vi "Main.vi"() -> ()   [LabVIEW 2010]
uses:
  Ctrls/Main_states.ctl
  Ctrls/Main_Msg_type.ctl
  Ctrls/NS3_commands.ctl
  Ctrls/ODSS_Msgs.ctl
  Vars/Comm_Vars.vi
panel:
  out "Time":timestamp caption="Simulation Time" format="%<%H:%M>T"
  out "V2":T1(graph) caption="Meter M2"
  out "Data":bool
  out "M2":string[][](table) caption="Monitor M2"
  out "M1":string[][](table) caption="Monitor M1"
  out "V1":T1(graph) caption="Meter M1"
  in  "ODSS Step":dbl[][](array[numeric])
  in  "NS3 Step":dbl[](array[numeric])
  out "Status":string
  in  "Stop":bool
  in  "Tasks":bool[](array[boolean])
  out "error out":errorcluster
  out "GB":picture
  in  "Quit":bool
  in  "start":bool
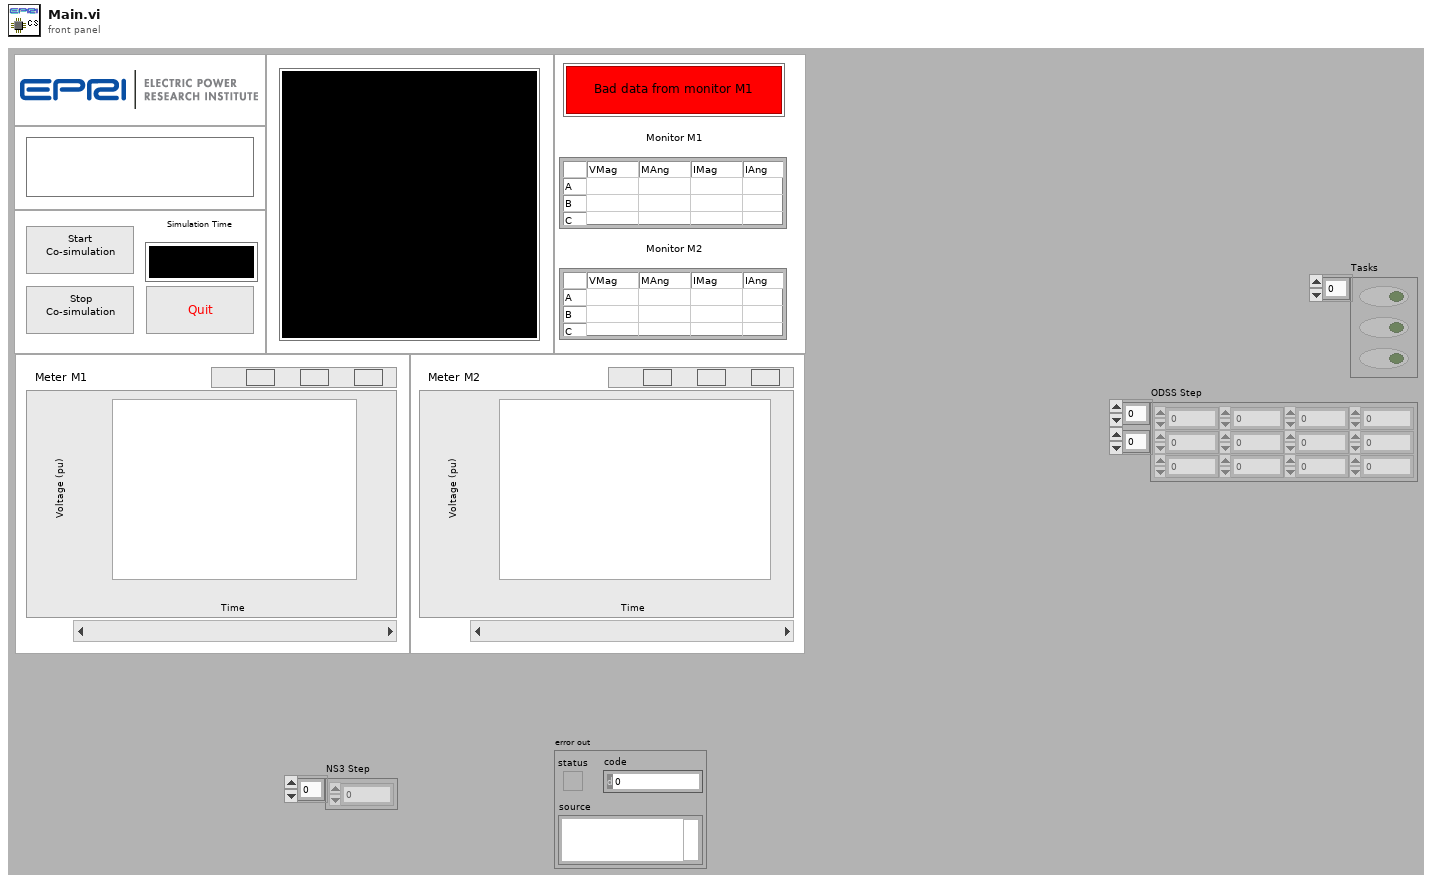
[diagram p1: front panel]
types:
  T1 = cluster{"Numeric":dbl, "Numeric":dbl, "Numeric":dbl}
  T2 = typedef "Main_Msg_type.ctl" = enum16{"Task end", "NS3 ready", "NS3 data", "Meter data", "exit"}
  T3 = typedef "Main_states.ctl" = enum16{"Init", "Launch NS3", "Launch OpenDSS", "Launch Meters", "Wait 4 user input", "Simulate", "Step in NS3", "Step in OpenDSS", "Publish Data", "Wait 4 Actors", "Kill actors", "Start exit routine", "Paint Meters", "End"}
  T4 = cluster{"Main_States":T3, "queue":refnum<queue>, "exit":bool, "Sim Started":bool, "Status":string, "next state":T3, "Bus info":cluster{"Bus Names":string[], "Bus Coords":cluster{i32, i32}[]}, "Circuit":picture, "Sim time":i32, "Paint":bool}
  T5 = cluster{"Rotate 90 deg":bool, "Flip Horizontally":bool, "Flip vertically":bool}
  T6 = cluster{"actor_name":string, "actor_type":string, "queue":refnum<queue>}[]
  T7 = typedef "NS3_commands.ctl" = enum16{"Init NS3 Sim", "Step in", "Exit"}
  T8 = typedef "ODSS_Msgs.ctl" = enum16{"Step in", "Exit", "Sim Time", "Set Working Dir"}
  T9 = cluster{"Numeric":dbl, "Numeric":dbl, "Numeric":dbl}[]
  T10 = cluster{"Bus Names":string[], "Bus Coords":cluster{i32, i32}[]}
  T11 = typedef "LVDateTimeRec.ctl" = cluster{"fractional second":dbl, "second":i32, "minute":i32, "hour":i32, "day of month":i32, "month":i32, "year":i32, "day of week":i32, "day of year":i32, "DST":i32}
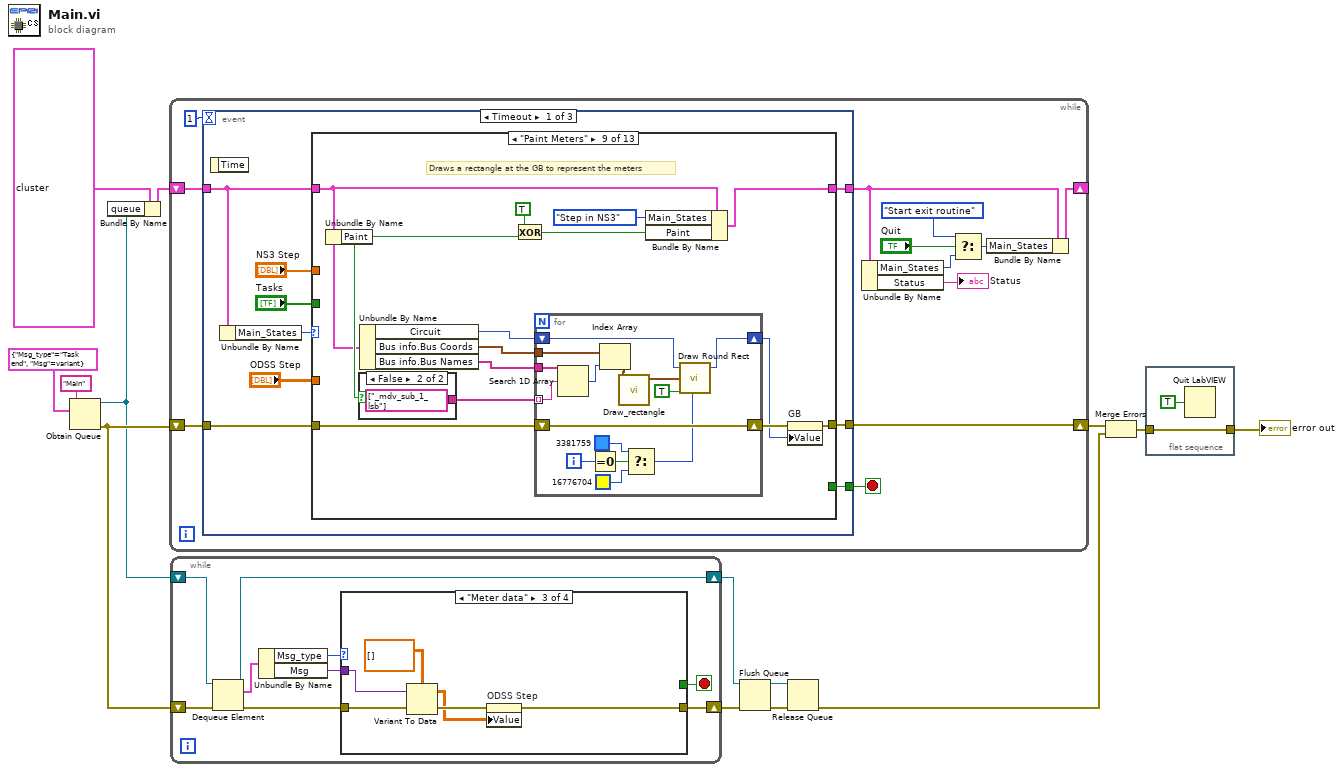
[diagram p0: block diagram]
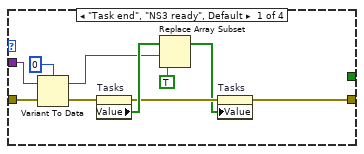
[diagram p2: hidden frame]
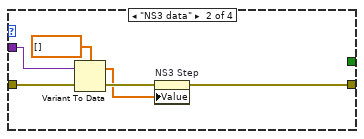
[diagram p3: hidden frame]
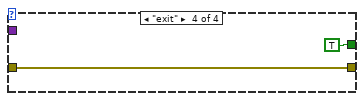
[diagram p4: hidden frame]
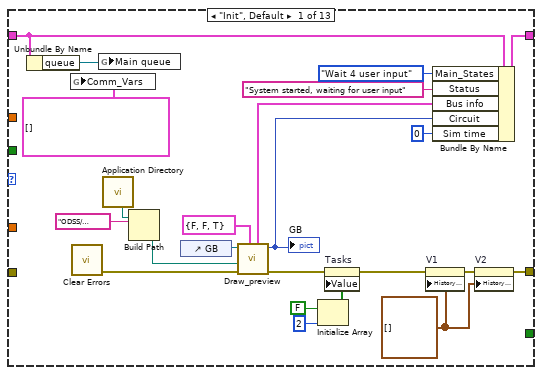
[diagram p5: hidden frame]
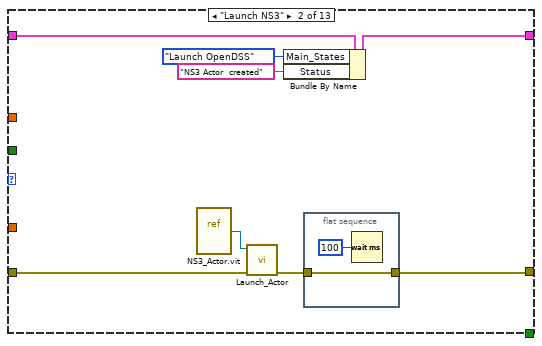
[diagram p6: hidden frame]
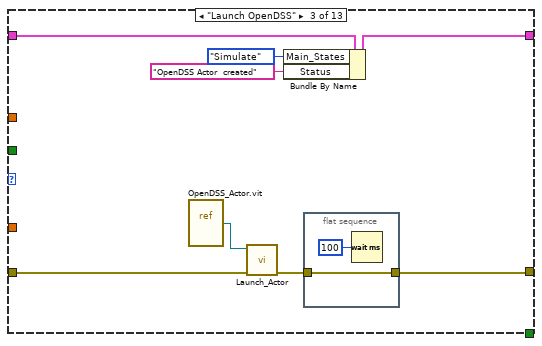
[diagram p7: hidden frame]
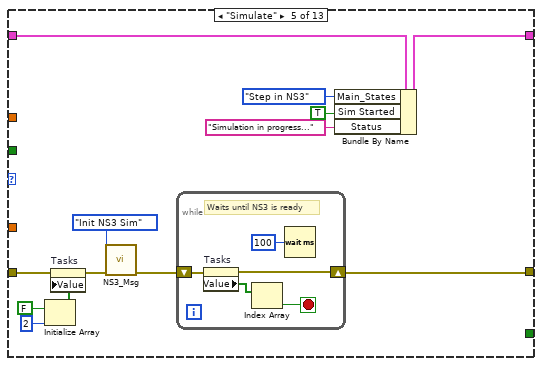
[diagram p9: hidden frame]
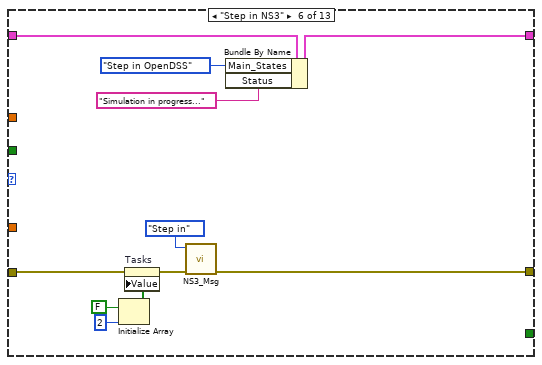
[diagram p10: hidden frame]
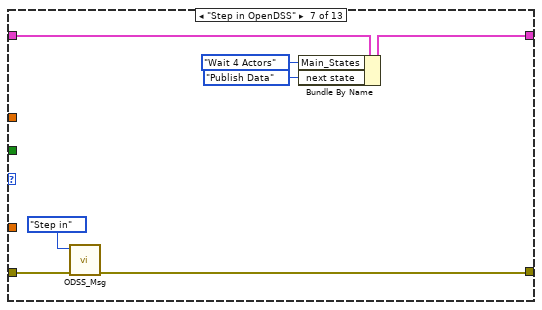
[diagram p11: hidden frame]
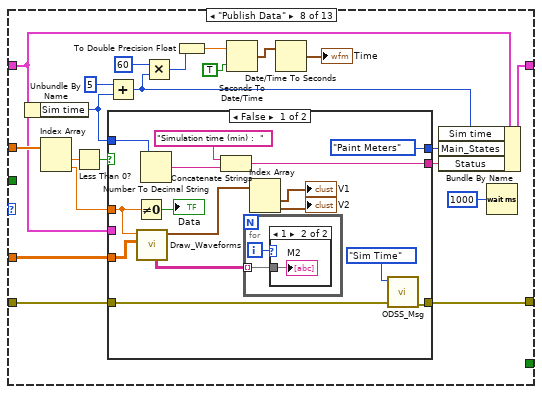
[diagram p12: hidden frame]
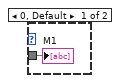
[diagram p13: hidden frame]
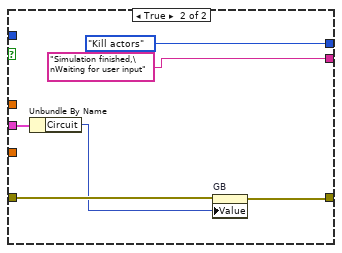
[diagram p14: hidden frame]
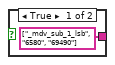
[diagram p15: hidden frame]
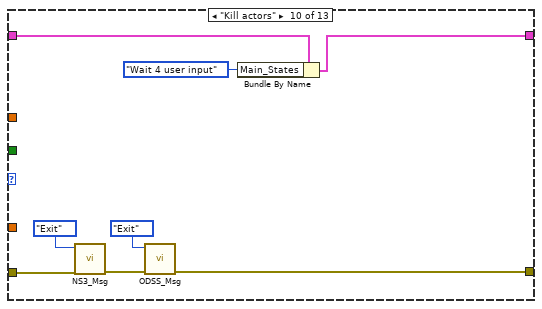
[diagram p16: hidden frame]
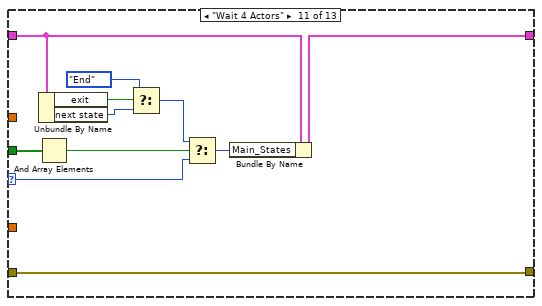
[diagram p17: hidden frame]
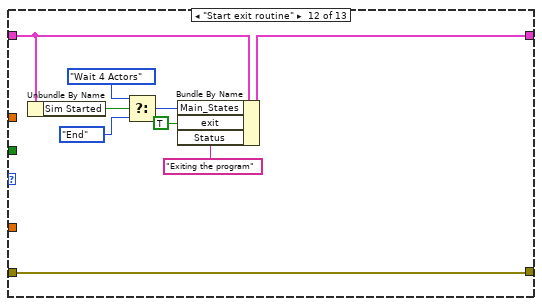
[diagram p18: hidden frame]
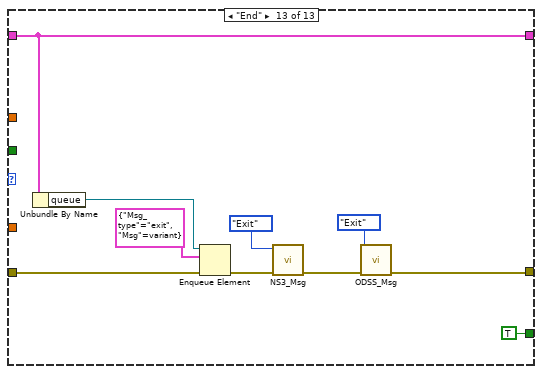
[diagram p19: hidden frame]
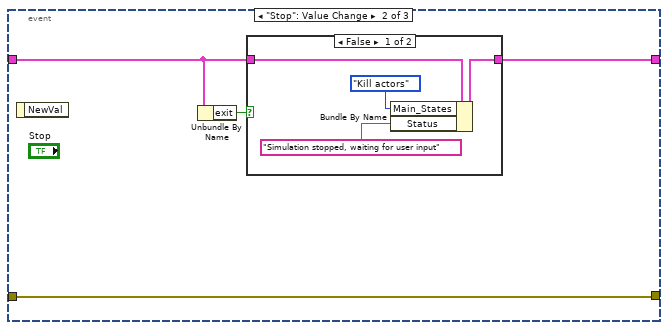
[diagram p20: hidden frame]
diagram:
  n1 = Obtain Queue(name (unnamed)="Main", element data type=cluster{"Msg_type":T2, "Msg":variant} {"Msg_type"=enum."Task end", "Msg"=variant}) -> (queue out=w10:refnum<queue>, error out=w12:errorcluster)  [unwired: 3 in, 1 out]
  n2 = Bundle By Name(cluster=T4 {"Main_States"=enum."Init", "queue"=refnum, "exit"=FALSE, "Sim Started"=FALSE, "Status"="", "next state"=enum."Init", "Bus info"={"Bus Names"=[], "Bus Coords"=[]}, "Circuit"=bytes[32946], "Sim time"=0, "Paint"=FALSE} ("variables"), "queue"=w10) -> (w3:T4)
  n3 = while {
    shift-right: [w16] -> _
    shift-left: w3 -> [w25]
    shift-right: [w23] -> w5
    shift-left: w12 -> [w22]
    stop <- w24 stop-if-true
    n4 = event shown="[0] Timeout" {
      selector: _ -> [_ _ _]
      dyn-events: _ -> [_ _ _]
      timeout: 1 -> [_ _ _]
      tunnel: w25 -> [w34 w234 w244]
      tunnel: [w33 w233 w242] -> w18
      tunnel: [w32 _ _] -> w24
      tunnel: [w27 w235 w245] -> w23
      tunnel: w22 -> [w31 w235 w245]
      event Timeout {
        n5 = event-data() -> ()  [unwired: 1 in, 1 out]
        n6 = Unbundle By Name(w34) -> ("Main_States"=w35:T3)
        n7 = case shown="\"Paint Meters\"" w35 {
          selector: w35 -> [_ _ _ _ _ _ _ _ _ _ w210 _ _]
          tunnel: w34 -> [w47 w65 w75 w80 w93 w105 w114 w117 w166 w201 w207 w219 w230]
          tunnel: [w56 w63 w73 w80 w92 w103 w113 w129 w175 w200 w208 w220 w230] -> w33
          tunnel: [_ _ _ _ _ _ _ _ _ _ _ _ TRUE] -> w32
          tunnel: w31 -> [_ w66 w76 w79 w86 w102 w116 w126 w169 w197 w202 w213 w227]
          tunnel: "Tasks" -> [_ _ _ _ _ _ _ _ _ _ w212 _ _]
          tunnel: "NS3 Step" -> [_ _ _ _ _ _ _ w128 _ _ _ _ _]
          tunnel: "ODSS Step" -> [_ _ _ _ _ _ _ w127 _ _ _ _ _]
          tunnel: [w38 w60 w70 w79 w81 w99 w110 w125 w171 w194 w202 w213 w223] -> w27
          frame "Init", Default {
            w37 = T9 [] ("History Data")
            n8 = Unbundle By Name(w47) -> ("queue"=w46:refnum<queue>)
            n9 = global write "Comm_Vars.vi" "Comm_Vars"(T6 [] ("Comm_Vars")) -> ()
            n10 = call <vilib>:"Clear Errors.vi"() -> ("error out"=w54:errorcluster)  [unwired: 7 in]
            n11 = global write "Comm_Vars.vi" "Main queue"(w46) -> ()
            n12 = call <vilib>:"Application Directory.vi"() -> ("Application Directory"=w52:path)
            n13 = Build Path(base path=w52, name or relative path="ODSS/BusCoords.dss") -> (appended path=w50:path)
            n14 = control-ref of="GB"() -> (w55:refnum<vi>)
            n15 = call "Draw_preview.vi"("Draw_ops"=T5 {"Rotate 90 deg"=FALSE, "Flip Horizontally"=FALSE, "Flip vertically"=TRUE}, "error in (no error)"=w54, "Path"=w50, "Picture ref"=w55) -> ("error out"=w45:errorcluster, "Picture out"=w41:picture, "Bus info"=w42:T10)  [unwired: 5 in]
            "GB" <- w41
            n16 = Initialize Array(FALSE, 2 ("dimension size")) -> (w44:bool[])
            n17 = property on="Tasks" class="Arr (strict)"(error in=w45, "Value"=w44) -> (error out=w36:errorcluster)  [unwired: 1 in, 1 out]
            n18 = property on="V1" class="WFChart (strict)"(error in=w36, "History Data"=w37) -> (error out=w39:errorcluster)  [unwired: 1 in, 1 out]
            n19 = Bundle By Name(cluster=w47, "Main_States"=Main_states."Wait 4 user input", "Status"="System started, waiting for user input", "Bus info"=w42, "Circuit"=w41, "Sim time"=0) -> (w56:T4)
            n20 = property on="V2" class="WFChart (strict)"(error in=w39, "History Data"=w37) -> (error out=w38:errorcluster)  [unwired: 1 in, 1 out]
          }
          frame "Launch NS3" {
            n21 = vi-ref "NS3_Actor.vit"() -> (w59:refnum<vi>)
            n22 = call "Launch_Actor.vi"("error in"=w66, "vi reference"=w59) -> ("error out"=w61:errorcluster)  [unwired: 9 in]
            n23 = Bundle By Name(cluster=w65, "Main_States"=Main_states."Launch OpenDSS", "Status"="NS3 Actor  created") -> (w63:T4)
            n24 = flat-sequence {
              tunnel: w61 -> [w68]
              tunnel: [w68] -> w60
              frame #0 {
                n25 = Wait (ms)(milliseconds to wait=u32 100) -> ()  [unwired: 1 out]
              }
            }
          }
          frame "Launch OpenDSS" {
            n26 = vi-ref "OpenDSS_Actor.vit"() -> (w69:refnum<vi>)
            n27 = call "Launch_Actor.vi"("error in"=w76, "vi reference"=w69) -> ("error out"=w71:errorcluster)  [unwired: 9 in]
            n28 = Bundle By Name(cluster=w75, "Main_States"=Main_states."Simulate", "Status"="OpenDSS Actor  created") -> (w73:T4)
            n29 = flat-sequence {
              tunnel: w71 -> [w78]
              tunnel: [w78] -> w70
              frame #0 {
                n30 = Wait (ms)(milliseconds to wait=u32 100) -> ()  [unwired: 1 out]
              }
            }
          }
          frame "Wait 4 user input" {
          }
          frame "Simulate" {
            n31 = Initialize Array(FALSE, 2 ("dimension size")) -> (w87:bool[])
            n32 = property on="Tasks" class="Arr (strict)"(error in=w86, "Value"=w87) -> (error out=w85:errorcluster)  [unwired: 1 in, 1 out]
            n33 = call "NS3_Msg.vi"("error in"=w85, "Msg"=NS3_commands."Init NS3 Sim") -> ("error out"=w82:errorcluster)  [unwired: 9 in]
            n34 = while {
              shift-right: [w97] -> w81
              shift-left: w82 -> [w98]
              stop <- w95 stop-if-true
              # "Waits until NS3 is ready"
              n35 = property on="Tasks" class="Arr (strict)"(error in=w98) -> (error out=w97:errorcluster, "Value"=w96:bool[])  [unwired: 1 in, 1 out]
              n36 = Index Array(array=w96) -> (element=w95:bool)  [unwired: 1 in]
              n37 = Wait (ms)(milliseconds to wait=u32 100) -> ()  [unwired: 1 out]
            }
            n38 = Bundle By Name(cluster=w93, "Main_States"=Main_states."Step in NS3", "Sim Started"=TRUE, "Status"="Simulation in progress...") -> (w92:T4)
          }
          frame "Step in NS3" {
            n39 = Initialize Array(FALSE, 2 ("dimension size")) -> (w106:bool[])
            n40 = property on="Tasks" class="Arr (strict)"(error in=w102, "Value"=w106) -> (error out=w101:errorcluster)  [unwired: 1 in, 1 out]
            n41 = call "NS3_Msg.vi"("error in"=w101, "Msg"=NS3_commands."Step in") -> ("error out"=w99:errorcluster)  [unwired: 9 in]
            n42 = Bundle By Name(cluster=w105, "Main_States"=Main_states."Step in OpenDSS", "Status"="Simulation in progress...") -> (w103:T4)
          }
          frame "Step in OpenDSS" {
            n43 = call "ODSS_Msg.vi"("error in"=w116, "Msg"=ODSS_Msgs."Step in") -> ("error out"=w110:errorcluster)  [unwired: 9 in]
            n44 = Bundle By Name(cluster=w114, "Main_States"=Main_states."Wait 4 Actors", "next state"=Main_states."Publish Data") -> (w113:T4)
          }
          frame "Publish Data" {
            n45 = Unbundle By Name(w117) -> ("Sim time"=w131:i32)
            n46 = Index Array(array=w128) -> (element #1=w135:dbl, element #2=w132:dbl)  [unwired: 2 in]
            n47 = Less Than 0?(x=w135) -> (x < 0?=w136:bool)
            n48 = Add(x=5, y=w131) -> (x+y=w124:i32)
            n49 = case shown="False" w136 {
              tunnel: w131 -> [w151 _]
              tunnel: [Main_states."Paint Meters" ("Main_States") Main_states."Kill actors" ("t")] -> w134
              tunnel: [w148 "Simulation finished,\nWaiting for user input" ("Status")] -> w133
              tunnel: w132 -> [w141 _]
              tunnel: w127 -> [w147 _]
              tunnel: w126 -> [w139 w160]
              tunnel: [w143 w159] -> w125
              tunnel: w117 -> [_ w158]
              frame False {
                n50 = Not Equal To 0?(x=w141) -> (x != 0?=→"Data":bool)
                n51 = call "Draw_Waveforms.vi"("ODSS Step"=w147, "Comm"=w141) -> ("Time M"=w146:T9, "Meter"=w140:string[][][])  [unwired: 8 in]
                n52 = Number To Decimal String(number=w151) -> (decimal integer string=w149:string)  [unwired: 1 in]
                n53 = Concatenate Strings("Simulation time (min) :  ", w149) -> (w148:string)
                n54 = for {
                  tunnel: w140 -> [w153] mode=indexing
                  i -> [w154]
                  n55 = case shown="1" w154 {
                    tunnel: w153 -> [w155 w156]
                    frame 0, Default {
                      "M1" <- w155
                    }
                    frame 1 {
                      "M2" <- w156
                    }
                  }
                }
                n56 = Index Array(array=w146) -> (element #1=→"V1":T1, element #2=→"V2":T1)  [unwired: 2 in]
                n57 = call "ODSS_Msg.vi"("error in"=w139, "Msg"=ODSS_Msgs."Sim Time") -> ("error out"=w143:errorcluster)  [unwired: 9 in]
              }
              frame True {
                n58 = Unbundle By Name(w158) -> ("Circuit"=w157:picture)
                n59 = property on="GB" class="Pict"(error in=w160, "Value"=w157) -> (error out=w159:errorcluster)  [unwired: 1 in, 1 out]
              }
            }
            n60 = Multiply(x=60, y=w124) -> (x*y=w122:i32)
            n61 = To Double Precision Float(number=w122) -> (double precision float=w121:dbl)
            n62 = Seconds To Date/Time(time stamp (now)=w121, to UTC (F)=TRUE) -> (date time rec=w120:T11)
            n63 = Date/Time To Seconds(2:w120) -> (0:→"Time":timestamp)  [unwired: 1 in]
            n64 = Bundle By Name(cluster=w117, "Sim time"=w124, "Main_States"=w134, "Status"=w133) -> (w129:T4)
            n65 = Wait (ms)(milliseconds to wait=u32 1000) -> ()  [unwired: 1 out]
          }
          frame "Paint Meters" {
            # "Draws a rectangle at the GB to represent the meters"
            n66 = Unbundle By Name(w166) -> ("Paint"=w172:bool)
            n67 = case shown="False" w172 {
              tunnel: [string[] ["_mdv_sub_1_lsb", "6580", "69490"] string[] ["_mdv_sub_1_lsb"]] -> w167
              frame True {
              }
              frame False {
              }
            }
            n68 = Unbundle By Name(w166) -> ("Circuit"=w163:picture, "Bus info.Bus Coords"=w164:cluster{i32, i32}[], "Bus info.Bus Names"=w165:string[])
            n69 = Exclusive Or(1:w172, 2:TRUE ("x")) -> (0:w173:bool)
            n70 = for {
              shift-right: [w188] -> w170
              shift-left: w169 -> [w188]
              tunnel: w165 -> [w191]
              tunnel: w164 -> [w190]
              shift-right: [w186] -> w168
              shift-left: w163 -> [w187]
              tunnel: w167 -> [w177] mode=indexing
              i -> [w182]
              n71 = Search 1D Array(1D array=w191, element=w177) -> (index of element=w189:i32)  [unwired: 1 in]
              n72 = Equal To 0?(x=w182) -> (x = 0?=w181:bool)
              n73 = Index Array(array=w190, index=w189) -> (element=w185:cluster{i32, i32})
              n74 = call "Draw_rectangle.vi"("Coords"=w185) -> ("rect"=w184:cluster{i32, i32, i32, i32})  [unwired: 10 in]
              n75 = Select(t=u32 3381759 ("color(black)"), s=w181, f=u32 16776704 ("color(black)")) -> (s? t:f=w178:u32)
              n76 = call <vilib>:"Draw Round Rect.vi"("picture"=w187, "rect"=w184, "fill?(F)"=TRUE, "color(black)"=w178) -> ("new picture"=w186:picture)  [unwired: 5 in]
            }
            n77 = Bundle By Name(cluster=w166, "Main_States"=Main_states."Step in NS3", "Paint"=w173) -> (w175:T4)
            n78 = property on="GB" class="Pict"(error in=w170, "Value"=w168) -> (error out=w171:errorcluster)  [unwired: 1 in, 1 out]
          }
          frame "Kill actors" {
            n79 = call "NS3_Msg.vi"("error in"=w197, "Msg"=NS3_commands."Exit") -> ("error out"=w195:errorcluster)  [unwired: 9 in]
            n80 = call "ODSS_Msg.vi"("error in"=w195, "Msg"=ODSS_Msgs."Exit") -> ("error out"=w194:errorcluster)  [unwired: 9 in]
            n81 = Bundle By Name(cluster=w201, "Main_States"=Main_states."Wait 4 user input") -> (w200:T4)
          }
          frame "Wait 4 Actors" {
            n82 = Unbundle By Name(w207) -> ("exit"=w206:bool, "next state"=w203:T3)
            n83 = And Array Elements(Boolean array=w212) -> (logical AND=w211:bool)
            n84 = Select(t=Main_states."End", s=w206, f=w203) -> (s? t:f=w204:T3)
            n85 = Select(t=w204, s=w211, f=w210) -> (s? t:f=w209:T3)
            n86 = Bundle By Name(cluster=w207, "Main_States"=w209) -> (w208:T4)
          }
          frame "Start exit routine" {
            n87 = Unbundle By Name(w219) -> ("Sim Started"=w218:bool)
            n88 = Select(t=Main_states."Wait 4 Actors" ("Main_States"), s=w218, f=Main_states."End" ("Main_States")) -> (s? t:f=w215:T3)
            n89 = Bundle By Name(cluster=w219, "Main_States"=w215, "exit"=TRUE, "Status"="Exiting the program") -> (w220:T4)
          }
          frame "End" {
            n90 = Unbundle By Name(w230) -> ("queue"=w229:refnum<queue>)
            n91 = Enqueue Element(queue=w229, element=cluster{"Msg_type":T2, "Msg":variant} {"Msg_type"=enum."exit", "Msg"=variant}, error in (no error)=w227) -> (error out=w225:errorcluster)  [unwired: 1 in, 2 out]
            n92 = call "NS3_Msg.vi"("error in"=w225, "Msg"=NS3_commands."Exit") -> ("error out"=w224:errorcluster)  [unwired: 9 in]
            n93 = call "ODSS_Msg.vi"("error in"=w224, "Msg"=ODSS_Msgs."Exit") -> ("error out"=w223:errorcluster)  [unwired: 9 in]
          }
        }
      }
      event "Stop": Value Change {
        n94 = event-data() -> ()  [unwired: 1 in, 1 out]
        n95 = Unbundle By Name(w234) -> ("exit"=w232:bool)
        n96 = case shown="False" w232 {
          tunnel: w234 -> [w239 w240]
          tunnel: [w238 w240] -> w233
          frame False {
            n97 = Bundle By Name(cluster=w239, "Main_States"=Main_states."Kill actors" ("f"), "Status"="Simulation stopped, waiting for user input") -> (w238:T4)
          }
          frame True {
          }
        }
      }
      event "start": Value Change {
        n98 = event-data() -> ()  [unwired: 1 in, 1 out]
        n99 = Bundle By Name(cluster=w244, "Main_States"=Main_states."Launch NS3", "Status"="Initializing simulation") -> (w242:T4)
      }
    }
    n100 = Unbundle By Name(w18) -> ("Main_States"=w20:T3, "Status"=→"Status":string)
    n101 = Select(t=Main_states."Start exit routine" ("Main_States"), s="Quit", f=w20) -> (s? t:f=w17:T3)
    n102 = Bundle By Name(cluster=w18, "Main_States"=w17) -> (w16:T4)
  }
  n103 = while {
    shift-right: [w249] -> w9
    shift-left: w12 -> [w254]
    shift-right: [w246] -> w8
    shift-left: w10 -> [w247]
    stop <- w248 stop-if-true
    n104 = Dequeue Element(queue=w247, error in (no error)=w254) -> (queue out=w246:refnum<queue>, element=w253:cluster{"Msg_type":T2, "Msg":variant}, error out=w250:errorcluster)  [unwired: 1 in, 1 out]
    n105 = Unbundle By Name(w253) -> ("Msg_type"=w252:T2, "Msg"=w251:variant)
    n106 = case shown="\"Meter data\"" w252 {
      tunnel: w251 -> [w263 w269 w275 _]
      tunnel: w250 -> [w264 w270 w276 w278]
      tunnel: [w255 w268 w274 w278] -> w249
      tunnel: [_ _ _ TRUE] -> w248
      frame "Task end", "NS3 ready", Default {
        n107 = Variant To Data(error in=w264, Variant=w263, type=0) -> (error out=w261:errorcluster, data=w259:i32)
        n108 = property on="Tasks" class="Arr (strict)"(error in=w261) -> (error out=w257:errorcluster, "Value"=w260:bool[])  [unwired: 1 in, 1 out]
        n109 = Replace Array Subset(array=w260, new element=TRUE ("new element/subarray"), index=w259) -> (w256:bool[])
        n110 = property on="Tasks" class="Arr (strict)"(error in=w257, "Value"=w256) -> (error out=w255:errorcluster)  [unwired: 1 in, 1 out]
      }
      frame "NS3 data" {
        n111 = Variant To Data(error in=w270, Variant=w269, type=dbl[] []) -> (error out=w267:errorcluster, data=w265:dbl[])
        n112 = property on="NS3 Step" class="Arr (strict)"(error in=w267, "Value"=w265) -> (error out=w268:errorcluster)  [unwired: 1 in, 1 out]
      }
      frame "Meter data" {
        n113 = Variant To Data(error in=w276, Variant=w275, type=dbl[][] []) -> (error out=w273:errorcluster, data=w271:dbl[][])
        n114 = property on="ODSS Step" class="Arr (strict)"(error in=w273, "Value"=w271) -> (error out=w274:errorcluster)  [unwired: 1 in, 1 out]
      }
      frame "exit" {
      }
    }
  }
  n115 = Flush Queue(queue=w8, error in (no error)=w9) -> (queue out=w6:refnum<queue>, error out=w7:errorcluster)  [unwired: 1 out]
  n116 = Release Queue(queue=w6, error in (no error)=w7) -> (error out=w4:errorcluster)  [unwired: 1 in, 2 out]
  n117 = Merge Errors(w5, w4) -> (w2:errorcluster)
  n118 = flat-sequence {
    tunnel: w2 -> [w280]
    tunnel: [w280] -> w1
    frame #0 {
      n119 = Quit LabVIEW(quit? (T)=TRUE) -> ()
    }
  }
  "error out" <- w1
